vi "Load-black-images.vi"(8 "error in":errorcluster, 11 "Data ref. in":refnum<data-value>) -> (0 "error IO":errorcluster, 3 "Data ref.":refnum<data-value>, 5 "Success?":bool)   [LabVIEW 2013, in "CameraVision.lvlib" / "CV-Main.lvclass"]
doc: "If any of the background corrections is enabled (background or hot-pixel correction), this function loads the black image files from the user provided path (in Processing>Correction) for each active camera. The function also checks whether the black image is the correct size (full image size) and in a supported image format (bmp, png, jpeg, jpeg2000, tiff). If an error is detected, a custom message is displayed."
uses:
  CV-Main.lvclass
  Correction/Background-correction.ctl
  CV-Main.lvclass/CV-Main.ctl
  Buffers/CV-Buffers.lvclass/CV-Buffers.ctl
  Correction/CV-Correction.lvclass/CV-Correction.ctl
  Configuration/CV-Configuration.lvclass/CV-Configuration.ctl
  UI/Popup-messages.ctl
  Correction/Read Background correction type.vi
  Correction/Read Background correction.vi
  Correction/Read Black image camera 1.vi
  Correction/Read Black image camera 2.vi
  Configuration/Read ROI width.vi
  Configuration/Read X-offsets.vi
  Configuration/Read ROI height.vi
  Configuration/Read Y-offsets.vi
  Read Config params.vi
  Read Correct params.vi
  Read Buffers.vi
  Buffers/Read Black image refs.vi
  Configuration/CV-Configuration.lvclass
  Correction/CV-Correction.lvclass
  Buffers/CV-Buffers.lvclass
  <vilib>/vision/NI_Vision_Development_Module.lvlib
  UI/CV-UI.lvclass
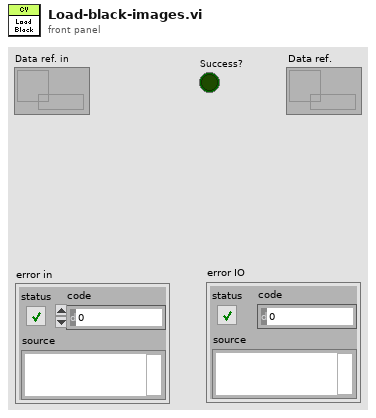
[diagram p1: front panel]
types:
  T1 = typedef "CameraVision.lvlib/CV-Correction.lvclass/Background-correction.ctl" = enum16{"Hardware", "Software"}
  T2 = typedef "CameraVision.lvlib/CV-UI.lvclass/Popup-messages.ctl" = enum16{"Error-Black image", "Error-Camera config file", "Error-Camera connect", "Error-Grabber init", "Error-Camera setting", "Error-Image offset", "Error-Image import", "Error-Settings file not exist", "Error-Timing source", "Conflict-Filters", "Conflict-Map", "Conflict-Framerate", "Conflict-Charact", "Conflict-Temperature field", "Conflict-Temperature value", "Conflict-Storage-Binary image", "Conflict-Storage-Corrected image", "Conflict-Storage-Map", "Conflict-Storage-Charact", "Conflict-Storage-Temperature field", "Conflict-Storage-Temperature value", "Warning-File exist", "Warning-Parameter reset", "Warning-User cancel", "Info-Images imported"}
  T3 = typedef "IMAQ Image.ctl" = refnum<image>
  T4 = typedef "CameraVision.lvlib/Correction.lvclass/Background-correction.ctl" = enum16{"Hardware", "Software"}
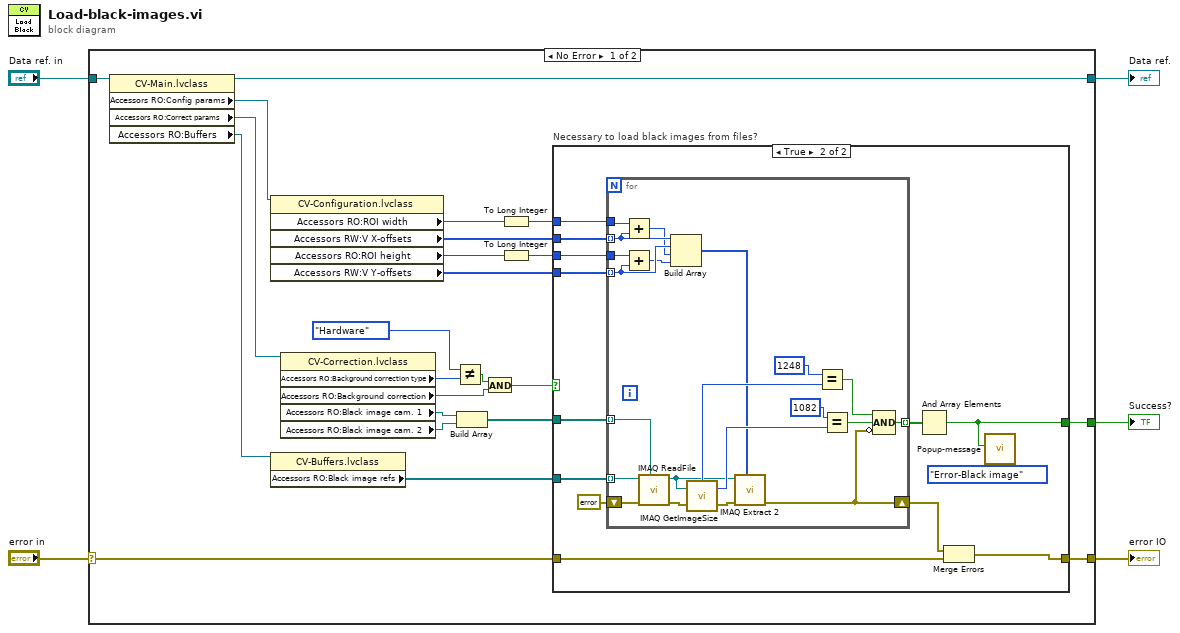
[diagram p0: block diagram]
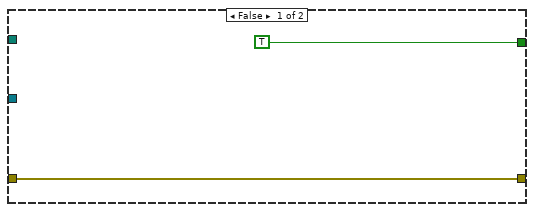
[diagram p2: hidden frame]
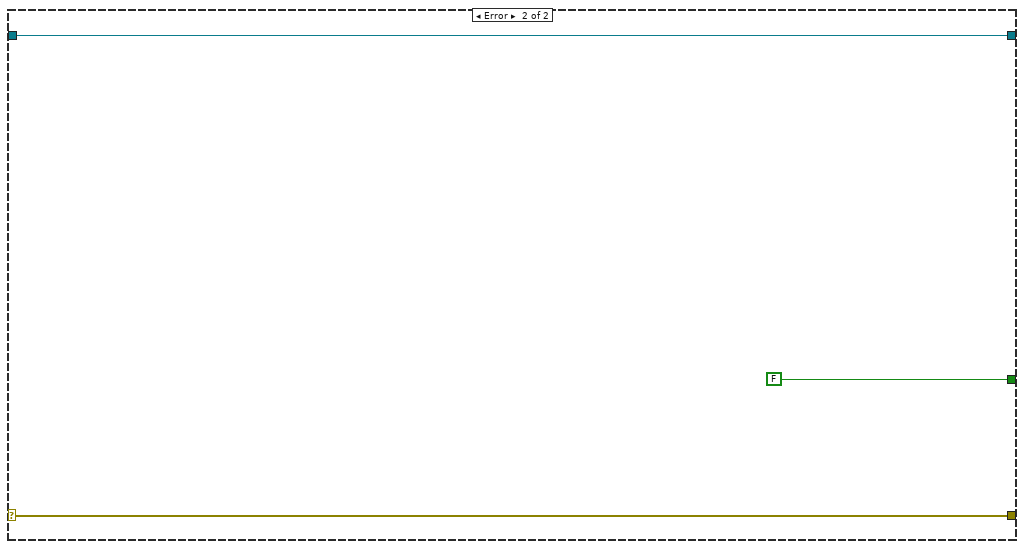
[diagram p3: hidden frame]
diagram:
  n1 = case shown="No Error" "error in" {
    selector: "error in" -> [w9 w67]
    tunnel: [w27 w67] -> w4
    tunnel: [w6 FALSE] -> w3
    tunnel: "Data ref. in" -> [w16 w65]
    tunnel: [w14 w65] -> w1
    frame No Error {
      n2 = property class="CV-Main.lvclass"(reference=w16) -> (reference out=w14:refnum<data-value>, "Accessors RO:Config params"=w12:refnum<data-value>, "Accessors RO:Correct params"=w11:refnum<data-value>, "Accessors RO:Buffers"=w13:refnum<class "CV-Buffers.lvclass">)  [unwired: 1 in, 1 out]
      n3 = property class="CV-Configuration.lvclass"(reference=w12) -> ("Accessors RO:ROI width"=w20:u32, "Accessors RW:V X-offsets"=w8:i32[], "Accessors RO:ROI height"=w19:u32, "Accessors RW:V Y-offsets"=w7:i32[])  [unwired: 1 in, 2 out]
      n4 = property class="CV-Buffers.lvclass"(reference=w13) -> ("Accessors RO:Black image refs"=w15:T3[])  [unwired: 1 in, 2 out]
      n5 = property class="CV-Correction.lvclass"(reference=w11) -> ("Accessors RO:Background correction type"=w25:T4, "Accessors RO:Background correction"=w22:bool, "Accessors RO:Black image cam. 1"=w10:path, "Accessors RO:Black image cam. 2"=w26:path)  [unwired: 1 in, 2 out]
      n6 = Not Equal?(x=Background-correction."Hardware", y=w25) -> (x != y?=w23:bool)
      n7 = Build Array(w10, w26) -> (w28:path[])
      n8 = And(x=w23, y=w22) -> (x .and. y?=w21:bool)
      n9 = To Long Integer(number=w20) -> (32bit integer=w17:i32)
      n10 = To Long Integer(number=w19) -> (32bit integer=w18:i32)
      n11 = case "Necessary to load black images from files?" shown="True" w21 {
        tunnel: w15 -> [_ w42]
        tunnel: w28 -> [_ w43]
        tunnel: [w29 w39] -> w27
        tunnel: [TRUE w31] -> w6
        tunnel: w8 -> [_ w37]
        tunnel: w7 -> [_ w36]
        tunnel: w9 -> [w29 w35]
        tunnel: w17 -> [_ w34]
        tunnel: w18 -> [_ w33]
        frame False {
        }
        frame True {
          n12 = for {
            tunnel: w43 -> [w64] mode=indexing
            tunnel: w42 -> [w63] mode=indexing
            shift-right: [w44] -> w40
            shift-left: errorcluster {"status"=FALSE, "code"=0, "source"=""} ("error constant") -> [w62]
            tunnel: [w54] -> w38 mode=indexing
            tunnel: w37 -> [w51] mode=indexing
            tunnel: w36 -> [w50] mode=indexing
            tunnel: w34 -> [w53]
            tunnel: w33 -> [w52]
            n13 = Add(x=w53, y=w51) -> (x+y=w49:i32)
            n14 = Add(x=w52, y=w50) -> (x+y=w48:i32)
            n15 = call "IMAQ ReadFile"("File Path"=w64, "error in (no error)"=w62, "Image"=w63) -> ("error out"=w61:errorcluster, "Image Out"=w46:T3)  [unwired: 4 in, 3 out]
            n16 = Build Array(w51, w50, w49, w48) -> (w47:i32[])
            n17 = call "IMAQ GetImageSize"("Image"=w46, "error in (no error)"=w61) -> ("Y Resolution"=w57:i32, "X Resolution"=w59:i32, "error out"=w45:errorcluster)  [unwired: 2 in]
            n18 = call "IMAQ Extract 2"("Optional Rectangle"=w47, "error in (no error)"=w45, "Image Src"=w46) -> ("error out"=w44:errorcluster)  [unwired: 7 in, 1 out]
            n19 = Equal?(x=1248, y=w59) -> (x = y?=w55:bool)
            n20 = Equal?(x=1082, y=w57) -> (x = y?=w56:bool)
            n21 = Compound Arithmetic op=AND(w55, w56, invert w44) -> (w54:bool)
          }
          n22 = And Array Elements(Boolean array=w38) -> (logical AND=w31:bool)
          n23 = Merge Errors(w40, w35) -> (w39:errorcluster)
          n24 = call "Popup-message.vi"("Message"=Popup-messages."Error-Black image", "Ignore?"=w31) -> ()  [unwired: 9 in, 1 out]
        }
      }
    }
    frame Error {
    }
  }
  "error IO" <- w4
  "Success?" <- w3
  "Data ref." <- w1
